vi "Open Ref from Path.vi"(8 "error in (no error)":errorcluster, 11 "VI Class Reference Control in":refnum<class "Class Reference Control.lvclass">) -> (0 "error out":errorcluster, 3 "VI Class Reference Control out":refnum<class "Class Reference Control.lvclass">)   [LabVIEW 2016, in "Class Reference Control.lvclass"]
uses:
  Class Reference Control.lvclass
  C:/Users/tblair/Documents/Git Projects/Drag and Drop VI Tool/Reference Control/Reference Control.lvclass
  Reference Control/Reference Control.lvclass/Reference Control.ctl
  Class Reference Control.lvclass/Class Reference Control.ctl
  Reference Control/Read Path Control Ref.vi
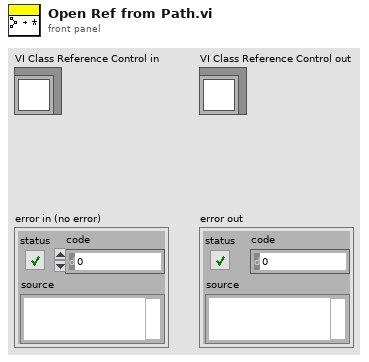
[diagram p1: front panel]
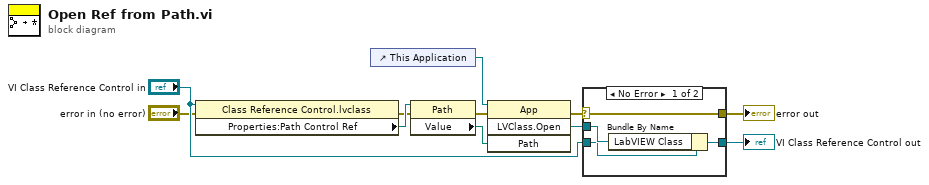
[diagram p0: block diagram]
diagram:
  n1 = property class="Class Reference Control.lvclass"(reference="VI Class Reference Control in", error in="error in (no error)") -> (error out=w10:errorcluster, "Properties:Path Control Ref"=w11:refnum<vi>)  [unwired: 1 out]
  n2 = control-ref of="This Application"() -> (w8:refnum<vi>)
  n3 = property on="Property Node" class="Path"(reference=w11, error in=w10) -> (error out=w5:errorcluster, "Value"=w7:path)  [unwired: 1 out]
  n4 = invoke class="App" method="LVClass.Open"(reference=w8, error in=w5, "Path"=w7) -> (error out=w4:errorcluster, "LVClass.Open"=w6:refnum<vi>)  [unwired: 1 in, 2 out]
  n5 = case shown="No Error" w4 {
    selector: w4 -> [w13 w17]
    tunnel: w6 -> [w15 _]
    tunnel: "VI Class Reference Control in" -> [w14 w16]
    tunnel: [w13 w17] -> w3
    tunnel: [w12 w16] -> w2
    frame No Error {
      n6 = Bundle By Name(cluster=w14, "LabVIEW Class"=w15) -> (w12:refnum<class "Class Reference Control.lvclass">)
    }
    frame Error {
    }
  }
  "error out" <- w3
  "VI Class Reference Control out" <- w2
